vi "Initialize.vi"(8 "Error In":errorcluster, 11 "VI Path":path) -> (0 "Error Out":errorcluster, 1 "Data Structures":T2, 2 "Action Queues":T3, 3 "Executable Configuration":T1)   [LabVIEW 2012]
uses:
  ActionQueues.ctl
  UIActionQueueElement.ctl
  UIAction.ctl
  HardwareActionQueueElement.ctl
  HardwareAction.ctl
  HeaterActionQueueElement.ctl
  HeaterAction.ctl
  MFCActionQueueElement.ctl
  MFCAction.ctl
  LogActionQueueElement.ctl
  LogAction.ctl
  DataStructures.ctl
  HardwareDisplayData.ctl
  HardwareLogData.ctl
  ExecutableConfiguration.ctl
  libs/LV-Utilities/LV-Utilities.lvlib
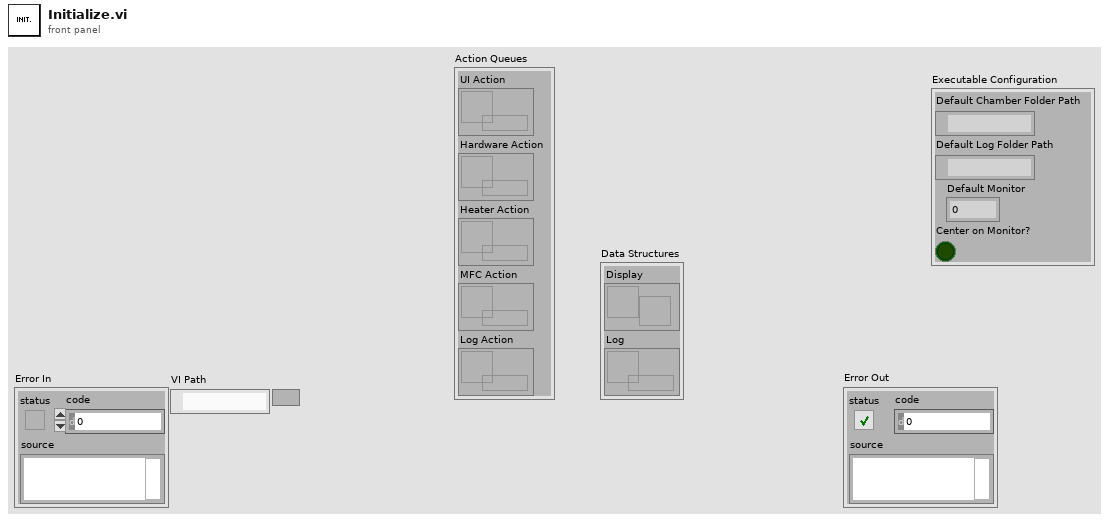
[diagram p1: front panel]
types:
  T1 = typedef "ExecutableConfiguration.ctl" = cluster{"Default Chamber Folder Path":path, "Default Log Folder Path":path, "Default Monitor":i32, "Center on Monitor?":bool}
  T2 = typedef "DataStructures.ctl" = cluster{"Display":refnum<notifier>, "Log":refnum<queue>}
  T3 = typedef "ActionQueues.ctl" = cluster{"UI Action":refnum<queue>, "Hardware Action":refnum<queue>, "Heater Action":refnum<queue>, "MFC Action":refnum<queue>, "Log Action":refnum<queue>}
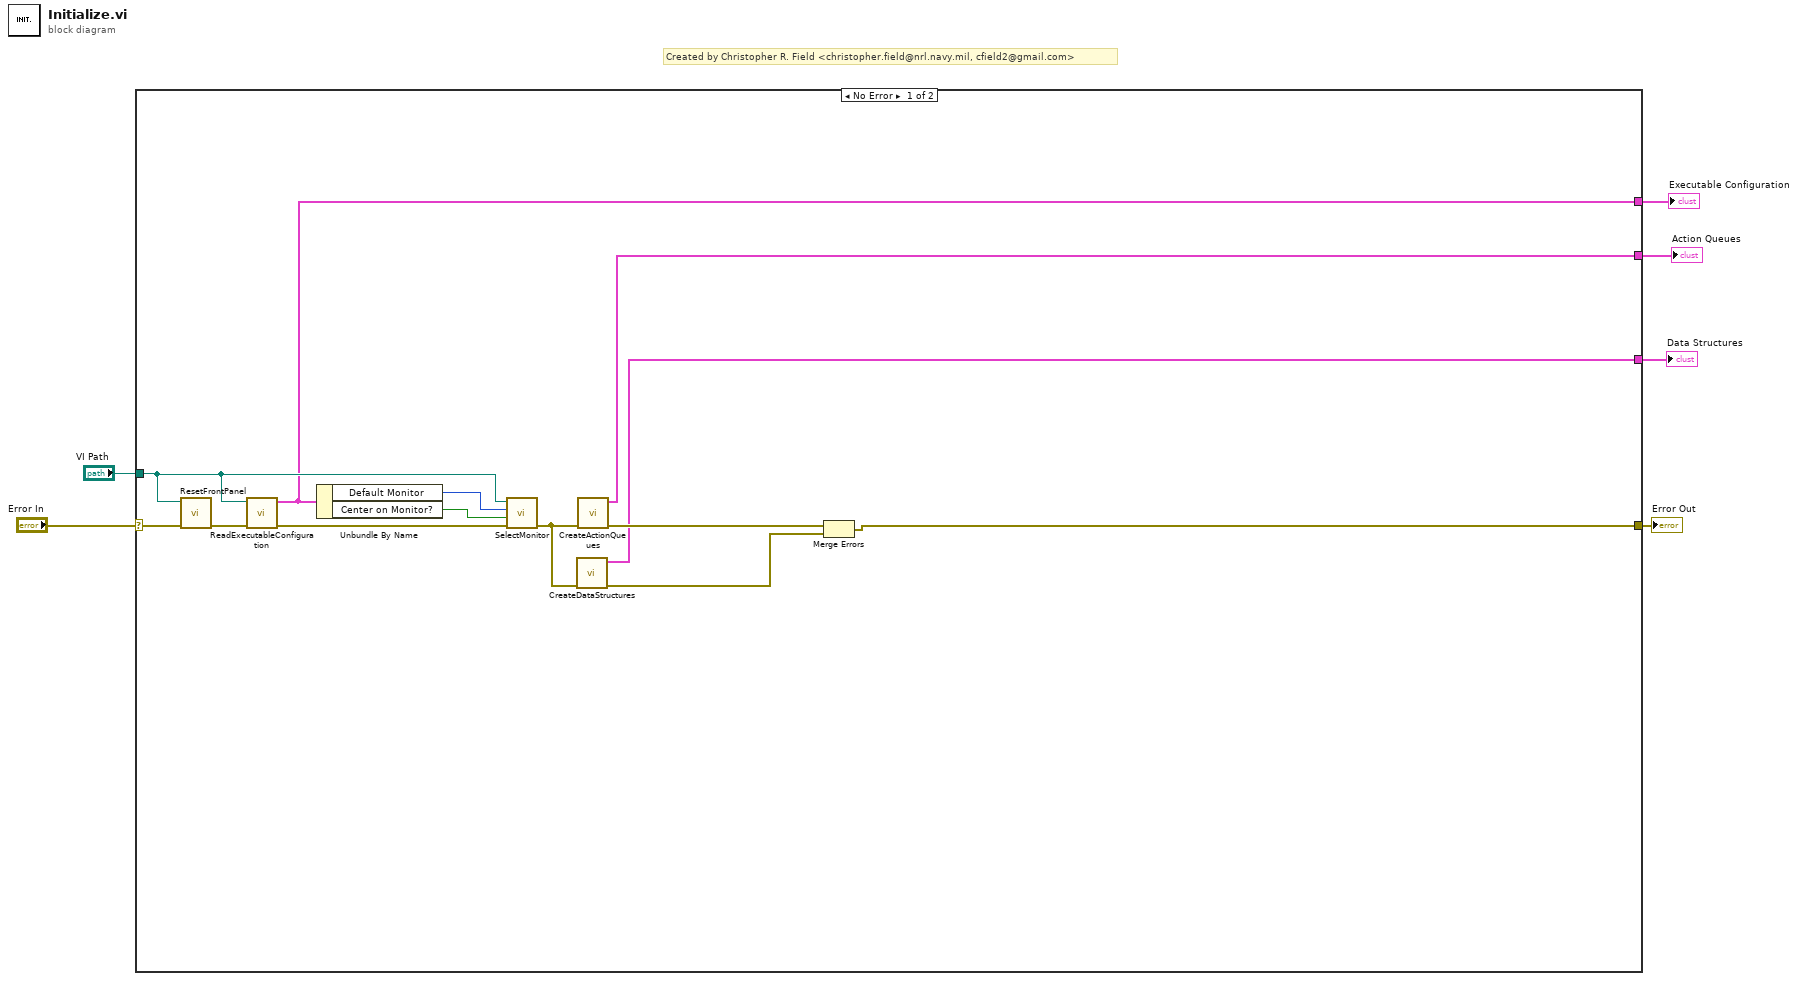
[diagram p0: block diagram]
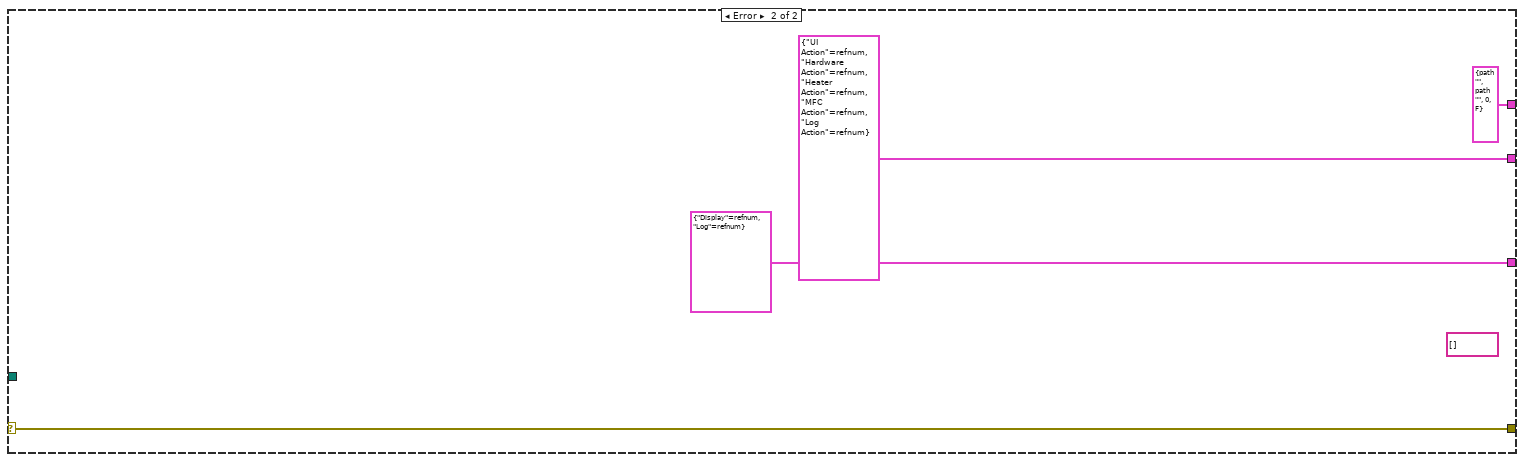
[diagram p2: hidden frame]
diagram:
  # "Created by Christopher R. Field <christopher.field@nrl.navy.mil, cfield2@gmail.com>"
  n1 = case shown="No Error" "Error In" {
    selector: "Error In" -> [w19 w23]
    tunnel: "VI Path" -> [w10 _]
    tunnel: [w15 w23] -> w4
    tunnel: [w18 T3 {"UI Action"=refnum, "Hardware Action"=refnum, "Heater Action"=refnum, "MFC Action"=refnum, "Log Action"=refnum} ("Action Queues")] -> w3
    tunnel: [w14 T2 {"Display"=refnum, "Log"=refnum} ("Data Structures")] -> w2
    tunnel: [w7 T1 {"Default Chamber Folder Path"=path "", "Default Log Folder Path"=path "", "Default Monitor"=0, "Center on Monitor?"=FALSE} ("Executable Configuration")] -> w1
    frame No Error {
      n2 = call "ResetFrontPanel.vi"("Error In"=w19, "VI Path"=w10) -> ("Error Out"=w12:errorcluster)  [unwired: 9 in]
      n3 = call "ReadExecutableConfiguration.vi"("Error In"=w12, "VI Path"=w10) -> ("Error Out"=w11:errorcluster, "Executable Configuration"=w7:T1)  [unwired: 8 in]
      n4 = Unbundle By Name(w7) -> ("Default Monitor"=w9:i32, "Center on Monitor?"=w8:bool)
      n5 = call "SelectMonitor.vi"("Error In"=w11, "Center?"=w8, "Monitor (0=primary)"=w9, "VI Path"=w10) -> ("Error out"=w13:errorcluster)  [unwired: 7 in]
      n6 = call "CreateDataStructures.vi"("Error In"=w13) -> ("Error Out"=w16:errorcluster, "Data Structures"=w14:T2)  [unwired: 9 in]
      n7 = call "CreateActionQueues.vi"("Error In"=w13) -> ("Error Out"=w17:errorcluster, "Action Queues"=w18:T3)  [unwired: 9 in]
      n8 = Merge Errors(w17, w16) -> (w15:errorcluster)
    }
    frame Error {
      (unwired) string[] [] ("VISA Resources")
    }
  }
  "Error Out" <- w4
  "Action Queues" <- w3
  "Data Structures" <- w2
  "Executable Configuration" <- w1
